vi "GetType.vi"(8 "error in (no error)":errorcluster, 11 "Configure Tranducer Type [TMP] Msg":refnum<class "Configure Tranducer Type [TMP] Msg.lvclass">) -> (0 "error out":errorcluster, 2 "Data Sample":variant, 3 "Configure Tranducer Type [TMP] Msg":refnum<class "Configure Tranducer Type [TMP] Msg.lvclass">)   [LabVIEW 2016, in "CS++DMM.lvlib" / "Configure Tranducer Type [TMP] Msg.lvclass"]
uses:
  Configure Tranducer Type [TMP] Msg.lvclass
  Configure Tranducer Type [TMP] Msg.lvclass/Configure Tranducer Type [TMP] Msg.ctl
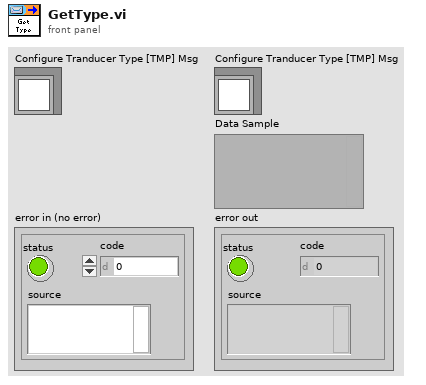
[diagram p1: front panel]
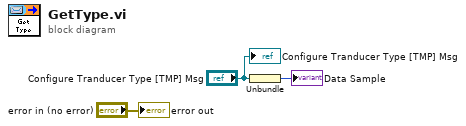
[diagram p0: block diagram]
diagram:
  n1 = Unbundle("Configure Tranducer Type [TMP] Msg") -> (→"Data Sample":i32)
  "error out" <- "error in (no error)"
  "Configure Tranducer Type [TMP] Msg" <- "Configure Tranducer Type [TMP] Msg"
